vi "OAT Torsional Vibration (Digital Tacho) (Waveform) (N Ch - N Settings).vi"(0 "digital tacho info":T2[](array[typedef]), 2 "pulse/revolution (1)":i32[](array[numeric]) min=1, 4 "torsional vibration units":enum16{"RPM", "deg/s", "rad/s"}(ring), 5 "error in (no error)":errorcluster, 8 "reset? (F)":bool, 10 "compensate geometric imperfection? (F)":bool, 11 "output interval [s]":dbl=0.001 min=0.0) -> (14 "torsional vibration signals":waveform(dbl)[](array[waveform]), 15 "speed profiles":T1[](array[typedef]) {"speed [RPM]" format="%.2f"; "time [s]" format="%.2f"}, 18 "unit labels":string[](array[string]), 19 "error out":errorcluster)   [LabVIEW 2017, in "SoundVib_Torsional.lvlib"]
doc: "Calculates torsional vibration signals from digital tachometer signals. This VI can return torsional vibration signals as either waveform signals or even-angle signals. Wire data to the <B>digital tacho info</B> input to determine the polymorphic instance to use or manually select the instance."
uses:
  <vilib>/addons/Sound and Vibration/Order Analysis/Torsional Vibration/SoundVib_Torsional.lvlib
  <vilib>/addons/Sound and Vibration/Order Analysis/Tach Process/SubVIs/digital tach info.ctl
  <vilib>/addons/Sound and Vibration/Order Analysis/Tach Process/SubVIs/speed profile.ctl
  <vilib>/addons/Sound and Vibration/Order Analysis/Tach Process/SoundVib_TachProcess.lvlib
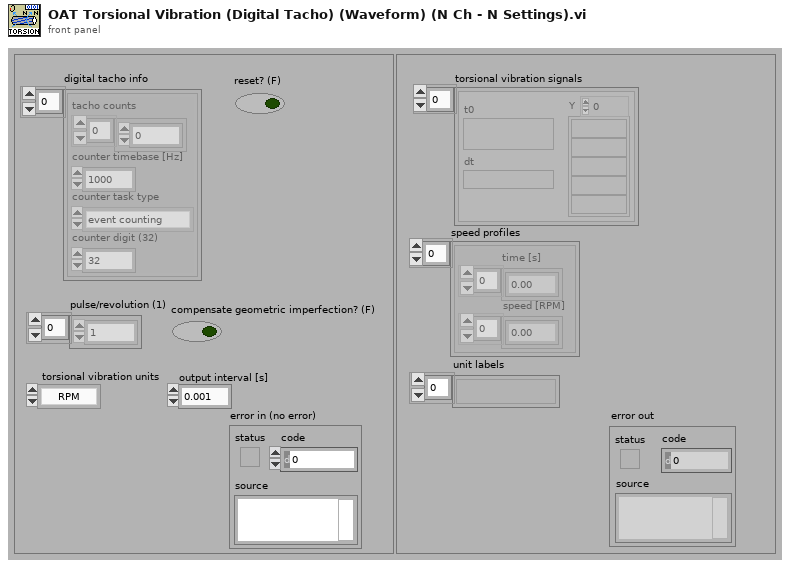
[diagram p1: front panel]
types:
  T1 = typedef "SoundVib_TachProcess.lvlib/speed profile.ctl" = cluster{"time [s]":dbl[], "speed [RPM]":dbl[]}
  T2 = typedef "SoundVib_TachProcess.lvlib/digital tach info.ctl" = cluster{"tacho counts":i64[], "counter timebase [Hz]":dbl, "counter task type":enum16{"period measurement", "event counting"}, "counter digit (32)":i32}
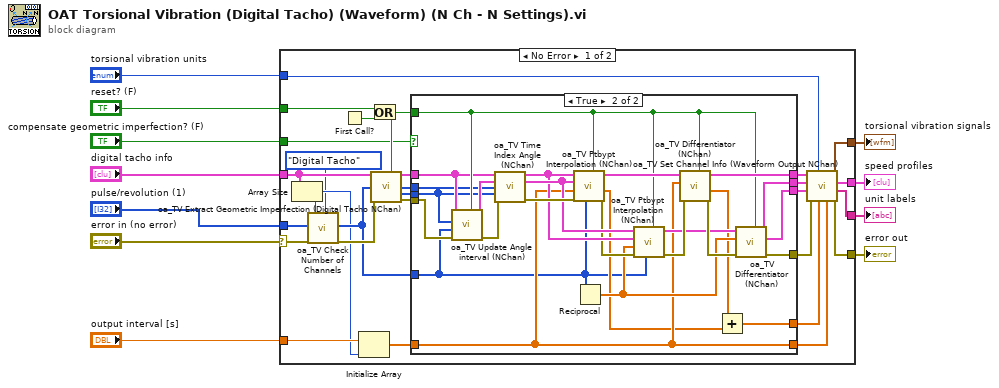
[diagram p0: block diagram]
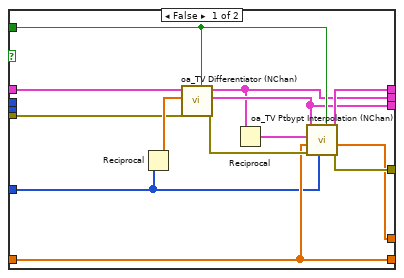
[diagram p2: hidden frame]
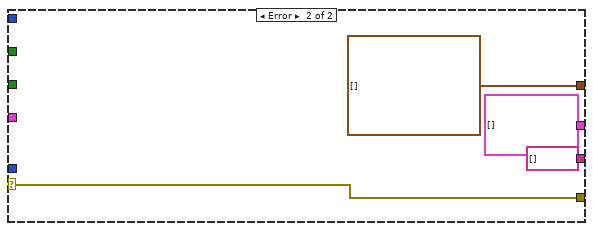
[diagram p3: hidden frame]
diagram:
  n1 = case shown="No Error" "error in (no error)" {
    selector: "error in (no error)" -> [w20 w81]
    tunnel: "compensate geometric imperfection? (F)" -> [w22 _]
    tunnel: "reset? (F)" -> [w36 _]
    tunnel: "digital tacho info" -> [w16 _]
    tunnel: "pulse/revolution (1)" -> [w17 _]
    tunnel: "torsional vibration units" -> [w27 _]
    tunnel: [w28 waveform(dbl)[] []] -> w7
    tunnel: [w31 w81] -> w6
    tunnel: [w26 T1[] [] ("speed profile")] -> w4
    tunnel: [w21 string[] [] ("unit labels")] -> w2
    tunnel: "output interval [s]" -> [w14 _]
    frame No Error {
      n2 = Array Size(array=w16) -> (size(s)=w13:i32)
      n3 = call <vilib>:"oa_TV Check Number of Channels.vi"("pulse/revolution (1)"=w17, "error in (no error)"=w20, "channel number"=w13, "tacho selection"=enum16{"Analog Tacho", "Digital Tacho"}."Digital Tacho") -> ("pulse/revolution out"=w18:i32[], "error out"=w19:errorcluster)  [unwired: 9 in, 5 out]
      n4 = First Call?() -> (First Call?: T/F=w37:bool)
      n5 = Initialize Array(w14, w13) -> (w15:dbl[])
      n6 = Or(x=w36, y=w37) -> (x .or. y?=w33:bool)
      n7 = call <vilib>:"oa_TV Extract Geometric Imperfection (Digital Tacho NChan).vi"("digital tacho info"=w16, "reset? (F)"=w33, "pulse/revolution"=w18, "error in (no error)"=w19) -> ("pulse positions"=w34:cluster{dbl[]}[], "revulotion"=w35:i32[], "revulotion index"=w38:i32[], "error out"=w39:errorcluster)  [unwired: 8 in]
      n8 = case shown="True" w22 {
        tunnel: w39 -> [w50 w56]
        tunnel: w38 -> [_ w55]
        tunnel: w35 -> [_ w57]
        tunnel: w34 -> [w52 w59]
        tunnel: w18 -> [w41 w54]
        tunnel: w33 -> [w49 w60]
        tunnel: [w43 w70] -> w32
        tunnel: [w48 w69] -> w30
        tunnel: [w40 w68] -> w29
        tunnel: [w42 w61] -> w25
        tunnel: w15 -> [w44 w64]
        tunnel: [w47 w65] -> w24
        tunnel: [w44 w64] -> w23
        frame False {
          n9 = Reciprocal(x=w41) -> (1/x=w51:dbl[])
          n10 = call <vilib>:"oa_TV Differentiator (NChan).vi"("reset? (False)"=w49, "error in (no error)"=w50, "delta X"=w51, "Y[n]"=w52) -> ("error out"=w45:errorcluster, "X[n]"=w47:cluster{dbl[]}[], "dY[n]/dX[n]"=w40:cluster{dbl[]}[])  [unwired: 4 in, 1 out]
          n11 = Reciprocal(x=w40) -> (1/x=w46:cluster{dbl[]}[])
          n12 = call <vilib>:"oa_TV Ptbypt Interpolation (NChan).vi"("reset? (F)"=w49, "buffer size"=w41, "error in (no error)"=w45, "dX"=w44, "Y"=w46, "X"=w47) -> ("error out"=w43:errorcluster, "X0"=w42:dbl[], "resampled Y"=w48:cluster{dbl[]}[])  [unwired: 2 in, 1 out]
        }
        frame True {
          n13 = call <vilib>:"oa_TV Update Angle interval (NChan).vi"("reset? (F)"=w60, "error in (no error)"=w56, "pulse/revolution"=w54, "revulotion index"=w55, "pulse position [s]"=w59) -> ("error out"=w53:errorcluster, "angle intervals"=w58:cluster{dbl[]}[])  [unwired: 5 in]
          n14 = call <vilib>:"oa_TV Time Index Angle (NChan).vi"("pulse positions"=w59, "angle intervals"=w58, "revulotion"=w57, "revulotion index"=w55, "error in (no error)"=w53) -> ("pulse positions"=w74:cluster{dbl[]}[], "angle"=w75:cluster{dbl[]}[], "error out"=w77:errorcluster)  [unwired: 8 in]
          n15 = call <vilib>:"oa_TV Ptbypt Interpolation (NChan).vi"("reset? (F)"=w60, "buffer size"=w54, "error in (no error)"=w77, "dX"=w64, "Y"=w75, "X"=w74) -> ("error out"=w73:errorcluster, "X0"=w62:dbl[], "resampled Y"=w76:cluster{dbl[]}[])  [unwired: 2 in, 1 out]
          n16 = Reciprocal(x=w54) -> (1/x=w67:dbl[])
          n17 = call <vilib>:"oa_TV Ptbypt Interpolation (NChan).vi"("reset? (F)"=w60, "buffer size"=w54, "error in (no error)"=w73, "dX"=w67, "Y"=w74, "X"=w75) -> ("error out"=w72:errorcluster, "resampled Y"=w66:cluster{dbl[]}[])  [unwired: 2 in, 2 out]
          n18 = call <vilib>:"oa_TV Differentiator (NChan).vi"("reset? (False)"=w60, "error in (no error)"=w72, "delta X"=w64, "Y[n]"=w76) -> ("error out"=w71:errorcluster, "Delay"=w63:dbl[], "dY[n]/dX[n]"=w69:cluster{dbl[]}[])  [unwired: 4 in, 1 out]
          n19 = Add(x=w63, y=w62) -> (x+y=w61:dbl[])
          n20 = call <vilib>:"oa_TV Differentiator (NChan).vi"("reset? (False)"=w60, "error in (no error)"=w71, "delta X"=w67, "Y[n]"=w66) -> ("error out"=w70:errorcluster, "X[n]"=w65:cluster{dbl[]}[], "dY[n]/dX[n]"=w68:cluster{dbl[]}[])  [unwired: 4 in, 1 out]
        }
      }
      n21 = call <vilib>:"oa_TV Set Channel Info (Waveform Output NChan).vi"("dt"=w23, "t0"=w25, "torisional vibration unit (RPM)"=w27, "error in (no error)"=w32, "pulse position"=w24, "seconds/revolution"=w29, "revolutions/minute"=w30) -> ("error out"=w31:errorcluster, "unit labels"=w21:string[], "speed profile"=w26:T1[], "torsional vibration"=w28:waveform(dbl)[])  [unwired: 1 in]
    }
    frame Error {
    }
  }
  "error out" <- w6
  "torsional vibration signals" <- w7
  "speed profiles" <- w4
  "unit labels" <- w2
